vi "DataFlowComplete_Name.vi"() -> (1 "message name":string)   [LabVIEW 2017, in "DataFlow.lvlib"]
uses:
  <vilib>/addons/InsightCM/Devices/Shared/Common/DataFlow/DataFlow.lvlib
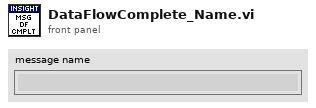
[diagram p1: front panel]
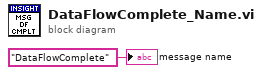
[diagram p0: block diagram]
diagram:
  "message name" <- "DataFlowComplete" ("ProcessName")
